vi "SimpleEval.vi"(11 "Input":string) -> (3 "Result":string)   [LabVIEW 2012]
uses:
  <vilib>/gmath/NI_Gmath.lvlib
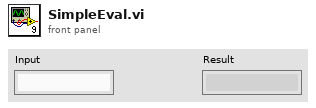
[diagram p1: front panel]
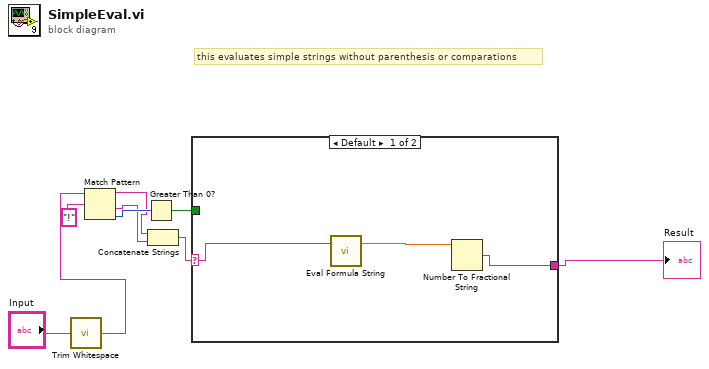
[diagram p0: block diagram]
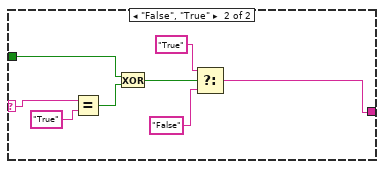
[diagram p2: hidden frame]
diagram:
  # "this evaluates simple strings without parenthesis or comparations"
  n1 = call <vilib>:"Trim Whitespace.vi"("string"="Input") -> ("trimmed string"=w5:string)  [unwired: 1 in]
  n2 = Match Pattern(string=w5, regular expression="!") -> (before substring=w3:string, after substring=w2:string, offset past match=w7:i32)  [unwired: 1 in, 1 out]
  n3 = Greater Than 0?(x=w7) -> (x > 0?=w4:bool)
  n4 = Concatenate Strings(w3, w2) -> (w1:string)
  n5 = case shown="Default" w1 {
    selector: w1 -> [w10 w20]
    tunnel: [w12 w13] -> w8
    tunnel: w4 -> [_ w17]
    frame Default {
      n6 = call <vilib>:"Eval Formula String.vi"("formula"=w10) -> ("y value"=w11:dbl)  [unwired: 1 in, 1 out]
      n7 = Number To Fractional String(number=w11) -> (F-format string=w12:string)  [unwired: 3 in]
    }
    frame "False", "True" {
      n8 = Equal?(x=w20, y="True") -> (x = y?=w18:bool)
      n9 = Exclusive Or(1:w18, 2:w17) -> (0:w16:bool)
      n10 = Select(t="True", s=w16, f="False") -> (s? t:f=w13:string)
    }
  }
  "Result" <- w8
